vi "Configure Network DNS.vi"(8 "error in (no error)":errorcluster, 10 "Network DNS (\"\")":string, 11 "VISA resource name":refnum<visa-resource-name>) -> (0 "error out":errorcluster, 3 "VISA resource name out":refnum<visa-resource-name>)   [LabVIEW 2020, in "Rohde&Schwarz CMXP Base.lvlib"]
doc: "Manually defines the DNS server IPv4 addresses to be used. A query returns the defined DNS addresses, irrespective of whether they have been specified manually or via DHCP.\n\nAttribute:\nRSCMXPBASE_ATTR_CONFIGURE_NETWORK_DNS\n\nRemote-control command:\nSYSTem:COMMunicate:NET:DNS"
uses:
  <instrlib>/Rohde&Schwarz CMXP Base/Rohde&Schwarz CMXP Base.lvlib
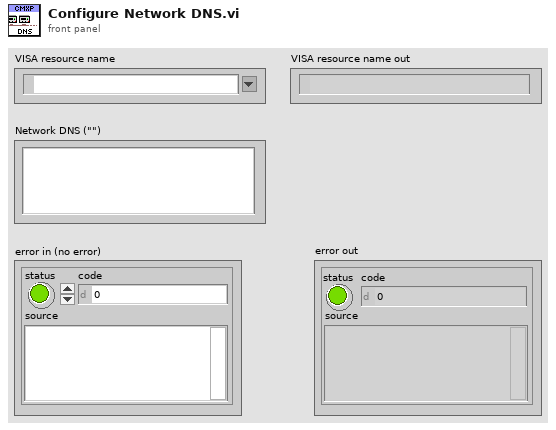
[diagram p1: front panel]
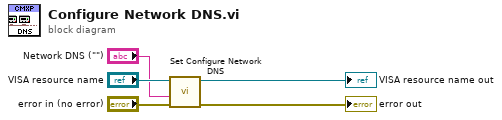
[diagram p0: block diagram]
diagram:
  n1 = call "Set Configure Network DNS"("error in (no error)"="error in (no error)", "Configure Network DNS ()"="Network DNS (\"\")", "instrument handle"="VISA resource name") -> ("error out"=→"error out":errorcluster, "instrument handle out"=→"VISA resource name out":refnum<visa-resource-name>)  [unwired: 7 in]
